vi "SetColor.vi"(8 "error in (no error)":errorcluster, 10 "Color":u32(colorbox), 11 "ColorGrayScale in":refnum<class "ColorGrayScale.lvclass">) -> (0 "error out":errorcluster, 3 "ColorGrayScale out":refnum<class "ColorGrayScale.lvclass">)   [LabVIEW 2021, in "Picture2D.lvlib" / "ColorGrayScale.lvclass"]
uses:
  ColorGrayScale.lvclass
  Color/Color.lvclass
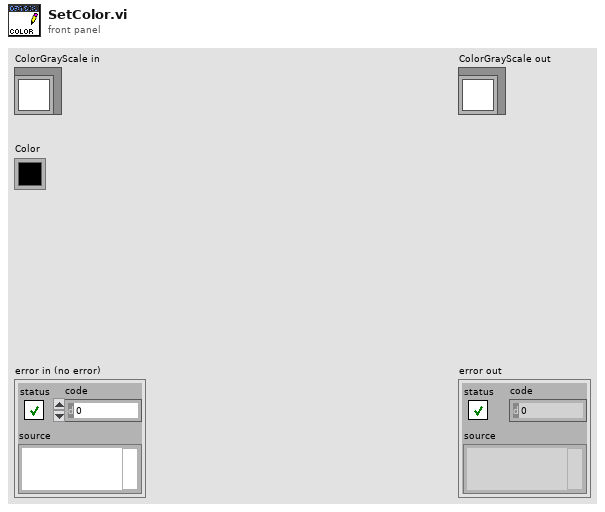
[diagram p1: front panel]
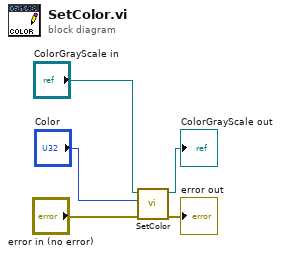
[diagram p0: block diagram]
diagram:
  n1 = call-parent "SetColor.vi"("error in (no error)"="error in (no error)", "Color"="Color", "Color in"="ColorGrayScale in") -> ("error out"=→"error out":errorcluster, "Color out"=→"ColorGrayScale out":refnum<class "ColorGrayScale.lvclass">)  [unwired: 7 in]
